vi "SPCConnect_HH.vi"(0 "error in (no error)":errorcluster) -> (2 "Error out":errorcluster)   [LabVIEW 2009]
uses:
  hhlib.dll
panel:
  in  "Case Constant\n(See Context Help)":bool
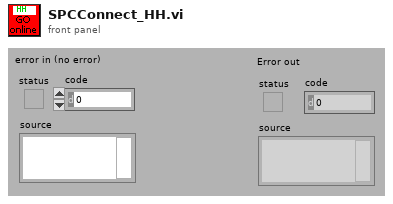
[diagram p1: front panel]
types:
  T1 = typedef "FIFOSettings.ctt" = cluster{"Measurement":cluster{"Binning (ms)":sgl, "External Trigger Condition":u16, "Stop Condition:":u16, "Stop Count":dbl, "Buffer Size (Photons)":u32, "No of Channels":u16, "Ext Latch Delay":i16}, "ADC":cluster{"Binning (HH)":i16, "Dither Range":i16, "Count Increment":i16, "Mode":u16}, "SYNC":cluster{"SYNC ZC Level (mV)":sgl, "SYNC Freq Divider":u16, "SYNC Holdoff (ps)":sgl, "SYNC Threshold (mV)":sgl}, "TAC":cluster{"TAC Range (ns)":sgl, "TAC Gain":i16, "TAC Offset (%)":sgl, "TAC Limit Low (%)":sgl, "TAC Limit High (%)":sgl}, "Ch 2":cluster{"Ch2 ZC Level (mV)":sgl, "Ch2 Holdoff (ps)":sgl, "Ch2 Threshold (mV)":sgl}, "Ch 3":cluster{"Ch3 ZC Level (mV)":sgl, "Ch3 Holdoff (ps)":sgl, "Ch3 Threshold (mV)":sgl}, "Ch 4":cluster{"Ch4 ZC Level (mV)":sgl, "Ch4 Holdoff (ps)":sgl, "Ch4 Threshold (mV)":sgl}, "Ch1":cluster{"Ch1 ZC Level (mV)":sgl, "Ch1 Holdoff (ps)":sgl, "Ch1 Threshold (mV)":sgl}}
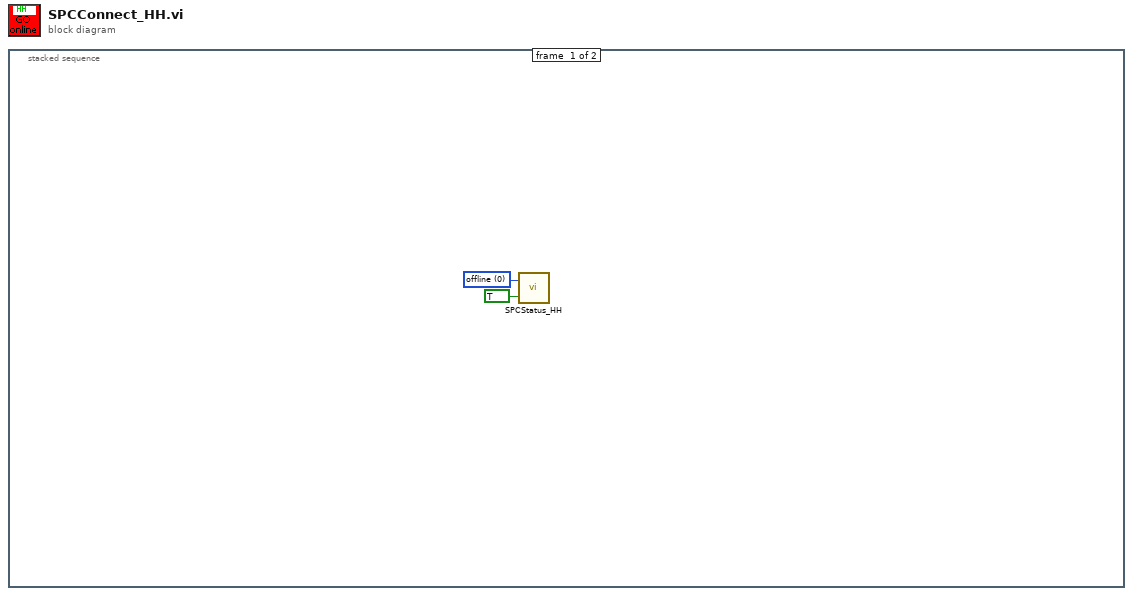
[diagram p0: block diagram]
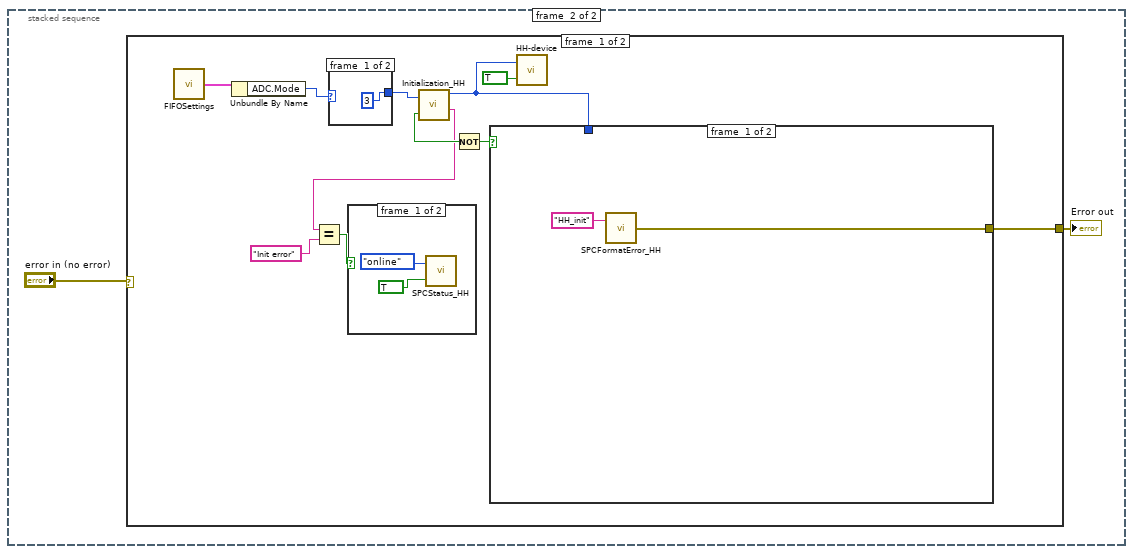
[diagram p2: hidden frame]
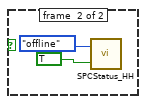
[diagram p3: hidden frame]
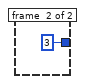
[diagram p4: hidden frame]
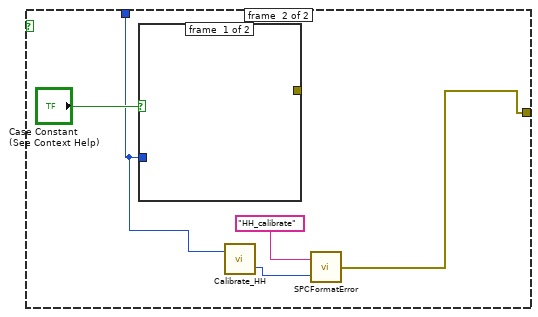
[diagram p5: hidden frame]
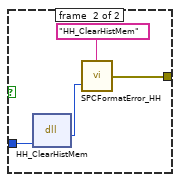
[diagram p6: hidden frame]
diagram:
  n1 = stacked-sequence {
    frame #0 {
      w2 = u16 0 items=["offline", "online", "busy"] ("Status code")
      n2 = call "SPCStatus_HH.vi"("Set/Get"=TRUE, "Status (input)"=w2) -> ()  [unwired: 1 out]
    }
    frame #1 {
      n3 = case shown="No Error" "error in (no error)" {
        selector: "error in (no error)" -> [_ w33]
        tunnel: [w15 w33] -> w3
        frame #0 {
          n4 = call "FIFOSettings.vi"() -> ("FIFO Settings(out)"=w14:T1)  [unwired: 2 in]
          n5 = Unbundle By Name(w14) -> ("ADC.Mode"=w11:u16)
          n6 = case shown="1, Default" w11 {
            tunnel: [3 3] -> w10
            frame #0 {
            }
            frame #1 {
            }
          }
          n7 = call "Initialization_HH.vi"("Mode"=w10) -> ("Initialisation Error"=w12:bool, "Deviceindex"=w9:i32, "Initialization Status"=w5:string)  [unwired: 2 out]
          n8 = Equal?(x=w5, y="Init error") -> (x = y?=w6:bool)
          n9 = case shown="True" w6 {
            frame #0 {
              n10 = call "SPCStatus_HH.vi"("Set/Get"=TRUE, "Status (input)"=enum16{"offline", "online", "busy"}."online") -> ()  [unwired: 1 out]
            }
            frame #1 {
              n11 = call "SPCStatus_HH.vi"("Set/Get"=TRUE, "Status (input)"=enum16{"offline", "online", "busy"}."offline") -> ()  [unwired: 1 out]
            }
          }
          n12 = Not(x=w12) -> (.not. x?=w13:bool)
          n13 = case shown="True" w13 {
            tunnel: [w22 w24] -> w15
            tunnel: w9 -> [_ w27]
            frame #0 {
              n14 = call "SPCFormatError_HH.vi"("Source"="HH_init") -> ("error out"=w22:errorcluster)  [unwired: 1 in]
            }
            frame #1 {
              n15 = case shown="True" "Case Constant\n(See Context Help)" {
                tunnel: w27 -> [_ w32]
                tunnel: [_ w29] -> _
                frame #0 {
                }
                frame #1 {
                  n16 = dll-call lib="C:/Programme/Anwendungen/DAQLinescan_HH/hhlib.dll" fn="HH_ClearHistMem"("devidx"=w32) -> (w31:i32)  [unwired: 4 in, 2 out]
                  n17 = call "SPCFormatError_HH.vi"("Error Code"=w31, "Source"="HH_ClearHistMem") -> ("error out"=w29:errorcluster)
                }
              }
              n18 = call "Calibrate_HH.vi"("Deviceindex"=w27) -> ("Returncode"=w25:i32)  [unwired: 1 in, 1 out]
              n19 = call "SPCFormatError.vi"("Error Code"=w25, "Source"="HH_calibrate") -> ("error out"=w24:errorcluster)
            }
          }
          n20 = call "HH-device.vi"("Set/Get"=TRUE, "Device (input)"=w9) -> ()  [unwired: 1 out]
        }
        frame #1 {
        }
      }
      "Error out" <- w3
    }
  }
